vi "Wrist main.vi"() -> ()   [LabVIEW 2018]
uses:
  <vilib>/Rock Robotics/WPI/ThirdParty/Phoenix-LabVIEW/Motor Controller/Controls/CTRE_Phoenix_MotorControl_FeedbackDevice.ctl
  <vilib>/Rock Robotics/WPI/ThirdParty/Phoenix-LabVIEW/Motor Controller/Controls/CTRE_Phoenix_MotorControl_ControlMode.ctl
  <vilib>/Rock Robotics/WPI/ThirdParty/Phoenix-LabVIEW/Motor Controller/Get/CTRE_Phoenix_MotorController_GetSelectedSensorData.vi
  Robot Global Data.vi
  <vilib>/Rock Robotics/Network Tables/NT Read Boolean.vi
  <vilib>/Rock Robotics/Network Tables/NT Write Number.vi
panel:
  in  "Tune Wrist":bool
  in  "reset pos":bool
  out "Wrist at home":bool
  in  "Disable?":bool
  in  "Wrist Selector":enum16{"Motion Magic", "Manual", "Disable"}(ring)
  in  "Output":dbl(slide) scale=-1.0..1.0
  in  "Setpoint":dbl
  in  "PIDF":T1={"P"=1.5, "I"=0.0005, "D"=0.0, "F"=0.0, "I zone"=0.0}
  out "Velocity (Raw Sensor Units per 100 ms)":i32
  out "Position (Raw Sensor Units)":i32
  in  "Acceleration":i32=220
  in  "Cruise Velocity":i32=200
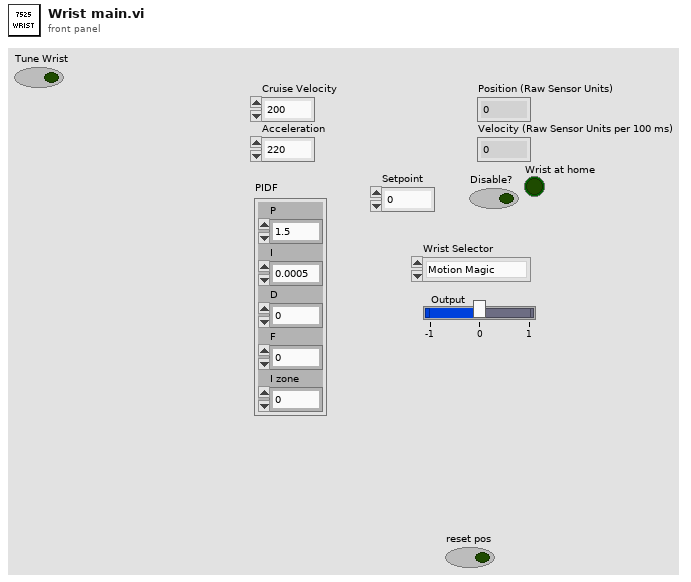
[diagram p1: front panel]
types:
  T1 = cluster{"P":dbl, "I":dbl, "D":dbl, "F":dbl, "I zone":dbl}
  T2 = typedef "CTRE_Phoenix_MotorControl_FeedbackDevice.ctl" = i8
  T3 = typedef "WPI_MotorControlDeviceRef.ctl" = cluster{"DeviceStatus":errorcluster, "Type":T4, "PWM":cluster{"PWM Channel":T5, "DeadBand":T6}, "CAN":cluster{"Device Number":u8, "SetOutput VI Ref":variant, "GetOutput VI Ref":variant, "Enable VI Ref":variant, "Disable VI Ref":variant, "Data":variant}, "Invert":bool, "DIO PWM":cluster{"PWM \"Enable\" Channel":T5, "DIOChannel":T7, "PWM Rate":dbl}}
  T4 = typedef "WPI_MotorControlType.ctl" = enum16{"PWM", "CAN", "DIO PWM"}
  T5 = typedef "FPGA_DIOPWMChannel.ctl" = enum8{"PWM 0", "PWM 1", "PWM 2", "PWM 3", "PWM 4", "PWM 5", "PWM 6", "PWM 7", "PWM 8", "PWM 9", "PWM MXP 0", "PWM MXP 1", "PWM MXP 2", "PWM MXP 3", "PWM MXP 4", "PWM MXP 5", "PWM MXP 6", "PWM MXP 7", "PWM MXP 8", "PWM MXP 9", "Invalid"}
  T6 = typedef "WPI_PWMDeadband.ctl" = cluster{"Name":string, "maxPositivePwm":i32, "minPositivePwm":i32, "centerPwm":i32, "maxNegativePwm":i32, "minNegativePwm":i32, "angularRange":u16}
  T7 = typedef "FPGA_DIOChannel.ctl" = enum8{"DIO 0", "DIO 1", "DIO 2", "DIO 3", "DIO 4", "DIO 5", "DIO 6", "DIO 7", "DIO 8", "DIO 9", "DIO MXP 0", "DIO MXP 1", "DIO MXP 2", "DIO MXP 3", "DIO MXP 4", "DIO MXP 5", "DIO MXP 6", "DIO MXP 7", "DIO MXP 8", "DIO MXP 9", "DIO MXP 10", "DIO MXP 11", "DIO MXP 12", "DIO MXP 13", "DIO MXP 14", "DIO MXP 15", "SPI Port CS1", "SPI Port CS2", "SPI Port CS3", "SPI Port MISO", "SPI Port MOSI", "Invalid"}
  T8 = typedef "CTRE_Phoenix_MotorControl_ControlMode.ctl" = u16
  T9 = typedef "WPI_SwitchDevRef.ctl" = cluster{"DevStatus":errorcluster, "DIO Channel":T7, "CntIndex":T10, "Normally Closed":bool}
  T10 = typedef "FPGA_CounterCtrSystemIndex.ctl" = enum8{"Ctr 0", "Ctr 1", "Ctr 2", "Ctr 3", "Ctr 4", "Ctr 5", "Ctr 6", "Ctr 7", "Invalid"}
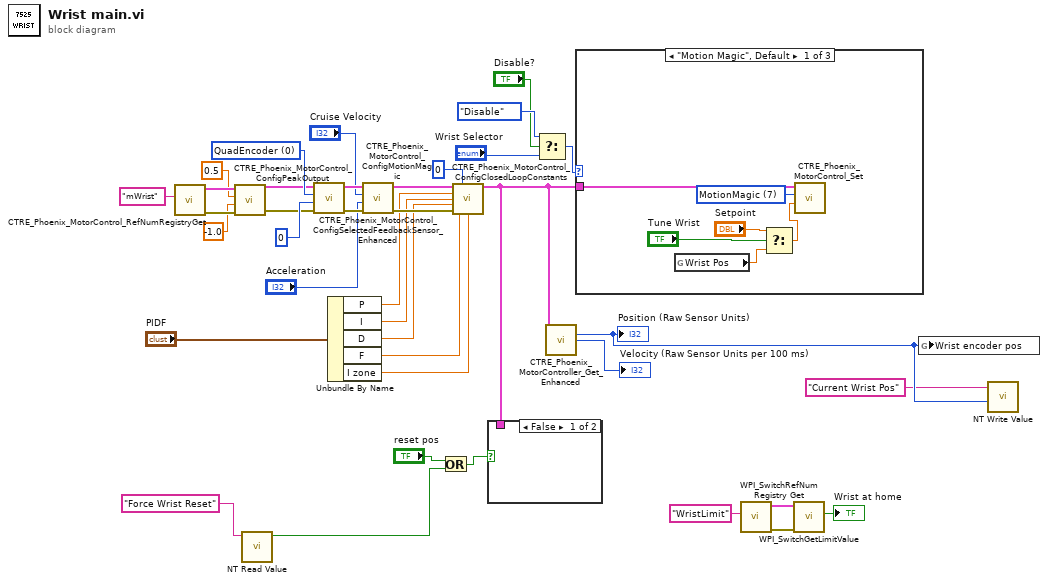
[diagram p0: block diagram]
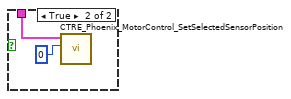
[diagram p2: hidden frame]
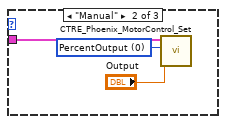
[diagram p3: hidden frame]
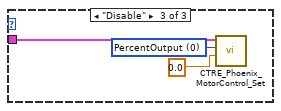
[diagram p4: hidden frame]
diagram:
  w33 = T2 0 items=["QuadEncoder"=0, "Analog"=2, "Tachometer"=4, "Pulse Width Encoded Position"=8, "Sensor Sum (S0 + S1)"=9, "Sensor Difference (D0 - D1)"=10, "Remote Source 0"=11, "Remote Source 1"=12, "Software Emulated"=15] ("Feedback Device")
  n1 = call <vilib>:"CTRE_Phoenix_MotorControl_RefNumRegistryGet.vi"("refnum name"="mWrist") -> ("error out"=w37:errorcluster, "PhoenixMotorControlDevRef"=w36:T3)  [unwired: 9 in]
  n2 = call <vilib>:"CTRE_Phoenix_MotorControl_ConfigPeakOutput.vi"("error in (no error)"=w37, "Reverse Peak Percent Output"=-1.0, "Forward Peak Percent Output"=0.5, "PhoenixMotorControlDevRef"=w36) -> ("error out"=w30:errorcluster, "PhoenixMotorControlDevRef"=w31:T3)  [unwired: 6 in]
  n3 = call-poly <vilib>:"NT Read Value.vi"("Name"="Force Wrist Reset") -> ("Boolean"=w3:bool)  [unwired: 9 in, 1 out]
  n4 = call <vilib>:"CTRE_Phoenix_MotorControl_ConfigSelectedFeedbackSensor_Enhanced.vi"("error in (no error)"=w30, "pidLoopIdx"=0, "Feedback Device"=w33, "PhoenixMotorControlDevRef"=w31) -> ("error out"=w29:errorcluster, "PhoenixMotorControlDevRef"=w28:T3)  [unwired: 6 in]
  n5 = Unbundle By Name("PIDF") -> ("P"=w20:dbl, "I"=w19:dbl, "D"=w18:dbl, "F"=w17:dbl, "I zone"=w16:dbl)
  n6 = call <vilib>:"CTRE_Phoenix_MotorControl_ConfigMotionMagic.vi"("error in (no error)"=w29, "Acceleration"="Acceleration", "Cruise Velocity"="Cruise Velocity", "PhoenixMotorControlDevRef"=w28) -> ("error out"=w23:errorcluster, "PhoenixMotorControlDevRef"=w24:T3)  [unwired: 6 in]
  n7 = Or(x="reset pos", y=w3) -> (x .or. y?=w6:bool)
  n8 = call <vilib>:"CTRE_Phoenix_MotorControl_ConfigClosedLoopConstants.vi"("PhoenixMotorControlDevRef"=w24, "slotIdx"=0, "P"=w20, "I"=w19, "D"=w18, "error in (no error)"=w23, "F"=w17, "I Zone"=w16) -> ("PhoenixMotorControlDevRef"=w7:T3)  [unwired: 6 in, 1 out]
  n9 = case shown="False" w6 {
    tunnel: w7 -> [_ w40]
    frame False {
    }
    frame True {
      n10 = call <vilib>:"CTRE_Phoenix_MotorControl_SetSelectedSensorPosition.vi"("New Sensor Position"=0, "PhoenixMotorControlDevRef"=w40) -> ()  [unwired: 8 in, 2 out]
    }
  }
  n11 = Select(t=enum16{"Motion Magic", "Manual", "Disable"}."Disable", s="Disable?", f="Wrist Selector") -> (s? t:f=w14:enum16{"Motion Magic", "Manual", "Disable"})
  n12 = call-poly <vilib>:"CTRE_Phoenix_MotorController_Get_Enhanced.vi"("PhoenixMotorControlDevRef"=w7) -> ("Position (Raw Sensor Units)"=w2:i32, "Velocity (Raw Sensor Units per 100 ms)"=→"Velocity (Raw Sensor Units per 100 ms)":i32)  [unwired: 11 in, 2 out]
  "Position (Raw Sensor Units)" <- w2
  n13 = case shown="\"Motion Magic\", Default" w14 {
    tunnel: w7 -> [w45 w49 w51]
    frame "Motion Magic", Default {
      w46 = T8 7 items=["PercentOutput"=0, "Position"=1, "Velocity"=2, "Current"=3, "Follower"=5, "MotionProfile"=6, "MotionMagic"=7, "MotionProfileArc"=10, "Disabled"=15] ("Control Mode")
      n14 = global read "Robot Global Data.vi" "Wrist Pos"() -> (w44:dbl)
      n15 = Select(t="Setpoint", s="Tune Wrist", f=w44) -> (s? t:f=w43:dbl)
      n16 = call <vilib>:"CTRE_Phoenix_MotorControl_Set.vi"("Output"=w43, "Control Mode"=w46, "PhoenixMotorControlDevRef"=w45) -> ()  [unwired: 7 in, 2 out]
    }
    frame "Manual" {
      w48 = T8 0 items=["PercentOutput"=0, "Position"=1, "Velocity"=2, "Current"=3, "Follower"=5, "MotionProfile"=6, "MotionMagic"=7, "MotionProfileArc"=10, "Disabled"=15] ("Control Mode")
      n17 = call <vilib>:"CTRE_Phoenix_MotorControl_Set.vi"("Output"="Output", "Control Mode"=w48, "PhoenixMotorControlDevRef"=w49) -> ()  [unwired: 7 in, 2 out]
    }
    frame "Disable" {
      w52 = T8 0 items=["PercentOutput"=0, "Position"=1, "Velocity"=2, "Current"=3, "Follower"=5, "MotionProfile"=6, "MotionMagic"=7, "MotionProfileArc"=10, "Disabled"=15] ("Control Mode")
      n18 = call <vilib>:"CTRE_Phoenix_MotorControl_Set.vi"("Output"=0.0, "Control Mode"=w52, "PhoenixMotorControlDevRef"=w51) -> ()  [unwired: 7 in, 2 out]
    }
  }
  n19 = call <vilib>:"WPI_SwitchRefNum Registry Get.vi"("refnum name"="WristLimit") -> ("error out"=w11:errorcluster, "SwitchDevRef"=w10:T9)  [unwired: 9 in]
  n20 = call <vilib>:"WPI_SwitchGetLimitValue.vi"("error in (no error)"=w11, "SwitchDevRef"=w10) -> ("Switch Pressed"=→"Wrist at home":bool)  [unwired: 7 in, 2 out]
  n21 = global write "Robot Global Data.vi" "Wrist encoder pos"(w2) -> ()
  n22 = call-poly <vilib>:"NT Write Value.vi"("Numeric"=w2, "Name"="Current Wrist Pos") -> ()  [unwired: 9 in, 1 out]
